vi "Register Objects.vi"(8 "error in":errorcluster, 9 "ID":string, 10 "Data":refnum<class "Data.lvclass">, 11 "Controller in":refnum<class "Controller.lvclass">) -> (0 "error out":errorcluster, 3 "Controller out":refnum<class "Controller.lvclass">)   [LabVIEW 2014, in "Controller.lvlib" / "Update Controller Data MSG.lvclass"]
doc: "Each data object is expected to register with using the Register Emmitter VI in the Controller Library. Once all have checked in, the Registration Complete flag is set in the Data Map DVR is set. At this point, we will write the header and begin writing to file.\n\nOn each update, the map is updated also for use by observers."
uses:
  Update Controller Data MSG.lvclass
  Controller.lvclass
  reusable/Data/Data.lvclass
  Controller.lvclass/Controller.ctl
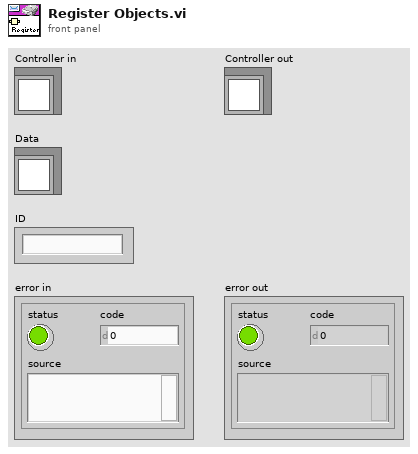
[diagram p1: front panel]
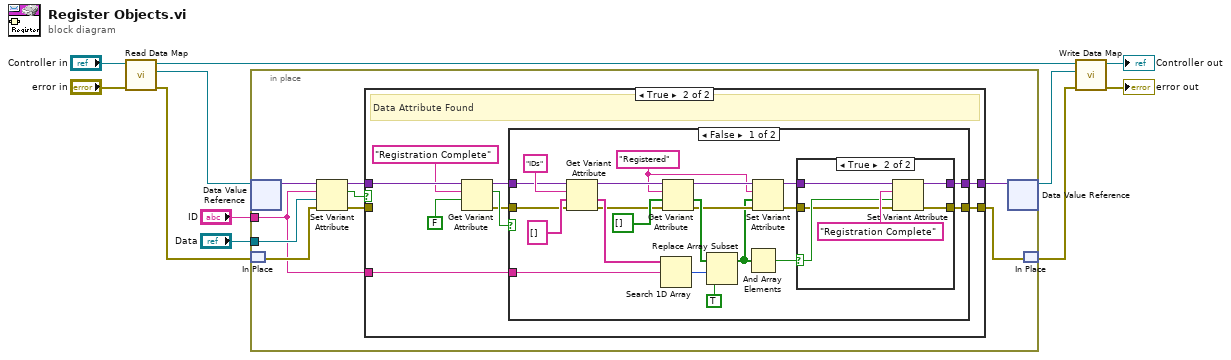
[diagram p0: block diagram]
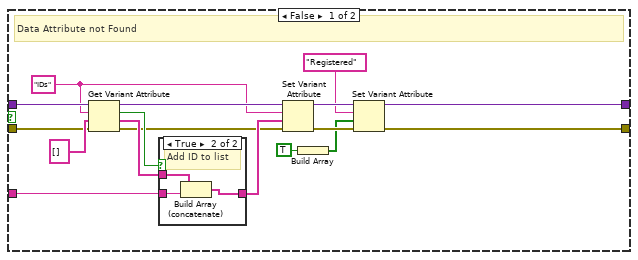
[diagram p2: hidden frame]
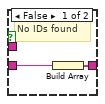
[diagram p3: hidden frame]
diagram:
  n1 = call "Read Data Map.vi"("error in"="error in", "Controller in"="Controller in") -> ("error out"=w4:errorcluster, "MAP DVR"=w2:refnum<data-value>, "Controller out"=w1:refnum<class "Controller.lvclass">)  [unwired: 7 in]
  n2 = in-place {
    in-place-border: "Data" -> [w18]
    in-place-border: "ID" -> [w14]
    n3 = in-place-dvr #1(w2) -> (w17:variant)  [unwired: 1 out]
    n4 = in-place-match #2(w4) -> (w15:errorcluster)
    n5 = Set Variant Attribute(Variant=w17, name=w14, value=w18, error in=w15) -> (Variant out=w20:variant, replaced=w19:bool, error out=w16:errorcluster)
    n6 = case shown="True" w19 {
      tunnel: w20 -> [w37 w49]
      tunnel: w14 -> [w31 w50]
      tunnel: [w25 w51] -> w12
      tunnel: w16 -> [w29 _]
      tunnel: [w24 w43] -> w13
      frame False {
        w34 = "IDs" ("name")
        # "Data Attribute not Found"
        n7 = Get Variant Attribute(Variant=w37, name=w34, default value (empty Variant)=string[] [], error in=w29) -> (duplicate Variant=w35:variant, found=w33:bool, value=w32:string[], error out=w28:errorcluster)
        n8 = case shown="True" w33 {
          tunnel: w32 -> [_ w42]
          tunnel: w31 -> [w39 w41]
          tunnel: [w38 w40] -> w30
          frame False {
            # "No IDs found"
            n9 = Build Array(w39) -> (w38:string[])
          }
          frame True {
            # "Add ID to list"
            n10 = Build Array (concatenate)(w42, w41) -> (w40:string[])
          }
        }
        n11 = Set Variant Attribute(Variant=w35, name=w34, value=w30, error in=w28) -> (Variant out=w27:variant, error out=w26:errorcluster)  [unwired: 1 out]
        n12 = Build Array(TRUE) -> (w21:bool[])
        n13 = Set Variant Attribute(Variant=w27, name="Registered", value=w21, error in=w26) -> (Variant out=w25:variant, error out=w24:errorcluster)  [unwired: 1 out]
      }
      frame True {
        # "Data Attribute Found"
        n14 = Get Variant Attribute(Variant=w49, name="Registration Complete", default value (empty Variant)=FALSE) -> (duplicate Variant=w45:variant, found=w46:bool, error out=w44:errorcluster)  [unwired: 1 in, 1 out]
        n15 = case shown="False" w46 {
          tunnel: [w55 w82] -> w51
          tunnel: w50 -> [w69 _]
          tunnel: w45 -> [w67 w82]
          tunnel: w44 -> [w66 w81]
          tunnel: [w53 w81] -> w43
          frame False {
            w58 = "Registered" ("name")
            n16 = Get Variant Attribute(Variant=w67, name="IDs", default value (empty Variant)=string[] [], error in=w66) -> (duplicate Variant=w68:variant, value=w70:string[], error out=w52:errorcluster)  [unwired: 1 out]
            n17 = Search 1D Array(1D array=w70, element=w69) -> (index of element=w63:i32)  [unwired: 1 in]
            n18 = Get Variant Attribute(Variant=w68, name=w58, default value (empty Variant)=bool[] [], error in=w52) -> (duplicate Variant=w61:variant, value=w64:bool[], error out=w60:errorcluster)  [unwired: 1 out]
            n19 = Replace Array Subset(array=w64, new element=TRUE ("new element/subarray"), index=w63) -> (w59:bool[])
            n20 = And Array Elements(Boolean array=w59) -> (logical AND=w56:bool)
            n21 = Set Variant Attribute(Variant=w61, name=w58, value=w59, error in=w60) -> (Variant out=w57:variant, error out=w54:errorcluster)  [unwired: 1 out]
            n22 = case shown="True" w56 {
              selector: w56 -> [_ w78]
              tunnel: w57 -> [w74 w80]
              tunnel: [w74 w77] -> w55
              tunnel: w54 -> [w73 w76]
              tunnel: [w73 w75] -> w53
              frame False {
              }
              frame True {
                n23 = Set Variant Attribute(Variant=w80, name="Registration Complete", value=w78, error in=w76) -> (Variant out=w77:variant, error out=w75:errorcluster)  [unwired: 1 out]
              }
            }
          }
          frame True {
          }
        }
      }
    }
    n24 = in-place-dvr #1(w12) -> (w3:refnum<data-value>)  [unwired: 1 out]
    n25 = in-place-match #2(w13) -> (w5:errorcluster)
  }
  n26 = call "Write Data Map.vi"("error in"=w5, "MAP DVR"=w3, "Controller in"=w1) -> ("error out"=→"error out":errorcluster, "Controller out"=→"Controller out":refnum<class "Controller.lvclass">)  [unwired: 7 in]
